vi "Actor Core.vi"(8 "error in":errorcluster, 11 "Hardware Interface Actor in":refnum<class "Hardware Interface Actor.lvclass">) -> (0 "error out":errorcluster, 3 "Actor out":refnum<class "Actor.lvclass">)   [LabVIEW 2026, in "Hardware Interface Actor.lvclass"]
doc: "<p>(<strong>Filename</strong>: <span class=\"dnl\">Actor Framework.lvlib:Actor.lvclass:Actor Core.vi</span>)</p>\n<p>Receives messages to the actor, reacts to them, and initiates any error handling that may shut the actor down.</p>\n<p>Descendant classes may override this VI to append parallel tasks for the actor to complete while it handles messages. Overrides use the <a href=\"nihelplauncher://docs/csh?context=lvcore_glang_udclass\">Call Parent Class Method</a> node.</p>"
uses:
  Hardware Interface Actor.lvclass
  C:/Program Files/National Instruments/LabVIEW 2026/vi.lib/ActorFramework/Actor/Actor.lvclass
  <vilib>/ActorFramework/Actor/Actor.lvclass
  <vilib>/ActorFramework/Actor/Actor.lvclass/Actor.ctl
  Hardware Interface Actor.lvclass/Hardware Interface Actor.ctl
  <vilib>/ActorFramework/Message Enqueuer/Message Enqueuer.lvclass/Message Enqueuer.ctl
  <vilib>/ActorFramework/Message Enqueuer/Enqueue.vi
  3_Full Actor/Tamagotchi Full Actor Messages/Feed Msg/Feed Msg.lvclass
  C:/Program Files/National Instruments/LabVIEW 2026/vi.lib/ActorFramework/Message/Message.lvclass
  3_Full Actor/Tamagotchi Full Actor Messages/Clean Msg/Clean Msg.lvclass
  3_Full Actor/Tamagotchi Full Actor Messages/Sleep Msg/Sleep Msg.lvclass
  3_Full Actor/Tamagotchi Full Actor Messages/Fixed Bug Msg/Fixed Bug Msg.lvclass
  3_Full Actor/Tamagotchi Full Actor Messages/Spaghetti Msg/Spaghetti Msg.lvclass
  3_Full Actor/Tamagotchi Full Actor Messages/Broken Arrow Msg/Broken Arrow Msg.lvclass
  <vilib>/ActorFramework/Message Priority Queue/Priority Enqueue.vi
  <vilib>/ActorFramework/Message Enqueuer/Message Enqueuer.lvclass
  C:/Users/dstark/OneDrive - Emerson/NI Connect 2026 Sessions/Intro to Actor Framework/4_A2A Comms/Hardware Interface Actor/Hardware Interface Actor.lvclass
panel:
  in  "stop":bool
  in  "Broken Arrow":bool
  in  "Spaghetti":bool
  in  "Fixed Bug":bool
  in  "Sleep":bool
  in  "Clean":bool
  in  "Feed":bool
  # "Stop calling actor to \nsto this VI"
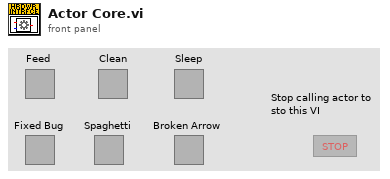
[diagram p1: front panel]
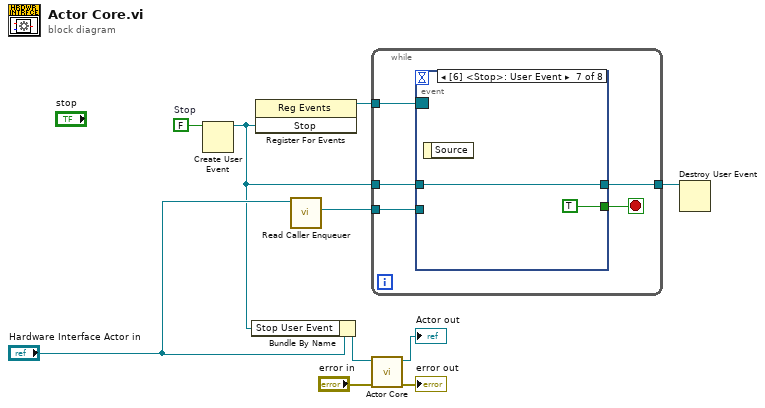
[diagram p0: block diagram]
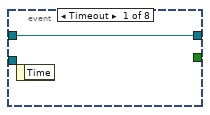
[diagram p2: hidden frame]
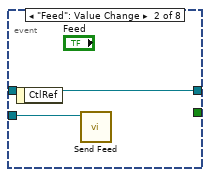
[diagram p3: hidden frame]
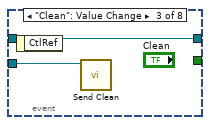
[diagram p4: hidden frame]
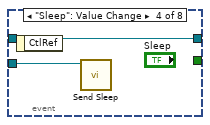
[diagram p5: hidden frame]
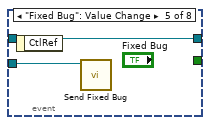
[diagram p6: hidden frame]
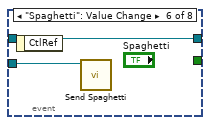
[diagram p7: hidden frame]
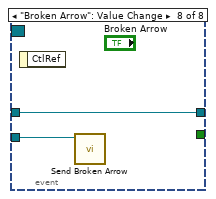
[diagram p8: hidden frame]
diagram:
  w5 = FALSE  # Stop
  n1 = Create User Event(user event datatype=w5) -> (user event=w1:refnum<user-event>)  [unwired: 1 in, 1 out]
  n2 = Bundle By Name(cluster="Hardware Interface Actor in", "Stop User Event"=w1) -> (w3:refnum<class "Hardware Interface Actor.lvclass">)
  n3 = register-events(w1) -> (reference out=w4:refnum<event-registration>)  [unwired: 2 in, 1 out]
  n4 = call <vilib>:"Read Caller Enqueuer.vi"("Actor"="Hardware Interface Actor in") -> ("Caller Enqueuer"=w6:refnum<class "Message Enqueuer.lvclass">)  [unwired: 10 in]
  n5 = while {
    tunnel: w6 -> [w15]
    tunnel: w4 -> [w13]
    tunnel: [w12] -> w2
    tunnel: w1 -> [w11]
    stop <- w14 stop-if-true
    n6 = event shown="[6] <Stop>: User Event" {
      selector: w13 -> [_ _ _ _ _ _ _ _]
      dyn-events: _ -> [_ _ _ _ _ _ _ _]
      timeout: _ -> [_ _ _ _ _ _ _ _]
      tunnel: w15 -> [_ w18 w20 w22 w24 w26 _ w30]
      tunnel: [_ _ _ _ _ _ TRUE ("stop") _] -> w14
      tunnel: [w16 w17 w19 w21 w23 w25 w28 w29] -> w12
      tunnel: w11 -> [w16 w17 w19 w21 w23 w25 w28 w29]
      event Timeout {
        n7 = event-data() -> ()  [unwired: 1 in, 1 out]
      }
      event "Feed": Value Change {
        n8 = event-data() -> ()  [unwired: 1 in, 1 out]
        n9 = call "Send Feed.vi"("Message Enqueuer"=w18) -> ()  [unwired: 9 in, 2 out]
      }
      event "Clean": Value Change {
        n10 = event-data() -> ()  [unwired: 1 in, 1 out]
        n11 = call "Send Clean.vi"("Message Enqueuer"=w20) -> ()  [unwired: 9 in, 2 out]
      }
      event "Sleep": Value Change {
        n12 = event-data() -> ()  [unwired: 1 in, 1 out]
        n13 = call "Send Sleep.vi"("Message Enqueuer"=w22) -> ()  [unwired: 9 in, 2 out]
      }
      event "Fixed Bug": Value Change {
        n14 = event-data() -> ()  [unwired: 1 in, 1 out]
        n15 = call "Send Fixed Bug.vi"("Message Enqueuer"=w24) -> ()  [unwired: 9 in, 2 out]
      }
      event "Spaghetti": Value Change {
        n16 = event-data() -> ()  [unwired: 1 in, 1 out]
        n17 = call "Send Spaghetti.vi"("Message Enqueuer"=w26) -> ()  [unwired: 9 in, 2 out]
      }
      event User Event {
        n18 = event-data() -> ()  [unwired: 1 in, 1 out]
      }
      event "Broken Arrow": Value Change {
        n19 = event-data() -> ()  [unwired: 1 in, 1 out]
        n20 = call "Send Broken Arrow.vi"("Message Enqueuer"=w30) -> ()  [unwired: 9 in, 2 out]
      }
    }
  }
  n21 = call-parent "Actor Core.vi"("error in"="error in", "Actor in"=w3) -> ("error out"=→"error out":errorcluster, "Actor out"=→"Actor out":refnum<class "Actor.lvclass">)  [unwired: 8 in]
  n22 = Destroy User Event(user event=w2) -> ()  [unwired: 1 in, 1 out]
